vi "Update Resistive Sim.vi"(8 "error in":errorcluster, 10 "Res Sim SPI command":T1, 11 "DMA FIFO ref":refnum<k20>) -> (0 "error out":errorcluster, 2 "FIU SPI command out":T1)   [LabVIEW 2014, in "SLSC configuration Engine.lvlib"]
uses:
  SLSC configuration Engine.lvlib
  Shared/Type Defs/Res Sim compiled.ctl
  <vilib>/NI Veristand/Custom Device API/Global Data Refs.vi
  <vilib>/Utility/error.llb/Error Cluster From Error Code.vi
  <vilib>/rvi/errors/niLvFpgaAdjustHostInterfaceError.vi
  <vilib>/rvi/interface/nirviMethod/nirviMethod.xnode
  <vilib>/NI Veristand/Custom Device API/Custom Device API.lvlib
  <vilib>/FPGAPlugInAG/Dynamic/niLvFpga_WriteFifo_Dynamic.vi
  <vilib>/rvi/errors/niLvFpgaMergeErrorWithErrorCode.vi
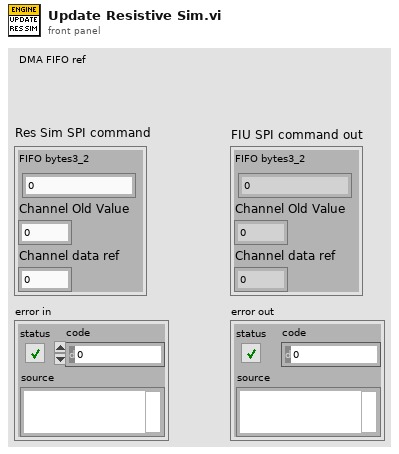
[diagram p1: front panel]
types:
  T1 = typedef "Res Sim compiled.ctl" = cluster{"FIFO bytes3_2":u16, "Channel Old Value":dbl, "Channel data ref":i32}
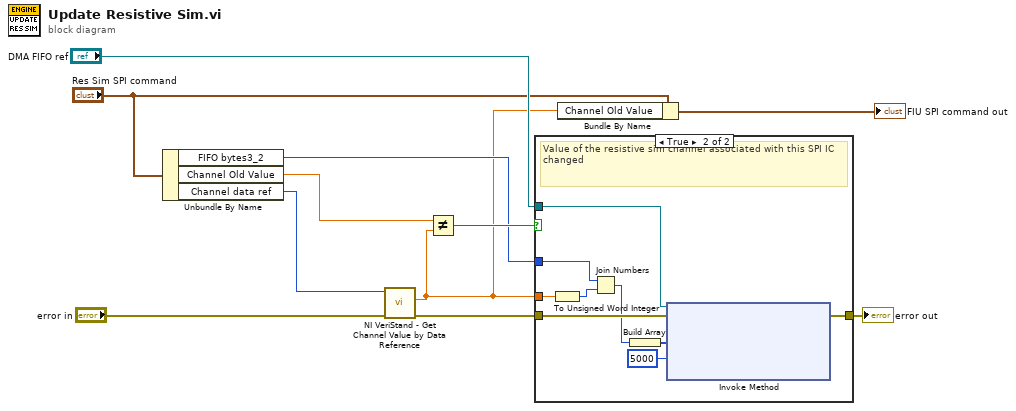
[diagram p0: block diagram]
diagram:
  n1 = Unbundle By Name("Res Sim SPI command") -> ("FIFO bytes3_2"=w7:u16, "Channel Old Value"=w9:dbl, "Channel data ref"=w11:i32)
  n2 = call <vilib>:"NI VeriStand - Get Channel Value by Data Reference.vi"("error in (no error)"="error in", "Data Reference in"=w11) -> ("error out"=w5:errorcluster, "Value"=w3:dbl)  [unwired: 8 out]
  n3 = Not Equal?(x=w9, y=w3) -> (x != y?=w8:bool)
  n4 = case shown="True" w8 {
    tunnel: w3 -> [_ w14]
    tunnel: w7 -> [_ w21]
    tunnel: "DMA FIFO ref" -> [_ w19]
    tunnel: w5 -> [w12 w20]
    tunnel: [w12 w15] -> w1
    frame False {
      # "No changes. Nothing to do here. Move on."
    }
    frame True {
      # "Value of the resistive sim channel associated with this SPI IC changed"
      n5 = To Unsigned Word Integer(number=w14) -> (unsigned 16bit integer=w13:u16)
      n6 = Join Numbers(hi=w21, lo=w13) -> ((hi.lo)=w18:u32)
      n7 = Build Array(w18) -> (w17:u32[])
      n8 = xnode "Invoke Method"("FPGA VI Reference In"=w19, "error in"=w20, "Data"=w17, "Timeout (ms)"=5000) -> ("error out"=w15:errorcluster)  [unwired: 2 out]
    }
  }
  "error out" <- w1
  n9 = Bundle By Name(cluster="Res Sim SPI command", "Channel Old Value"=w3) -> (→"FIU SPI command out":T1)
